vi "Shutdown.vi"(8 "Error In":errorcluster, 11 "libssh2-lv Shared Library":path=path "") -> (0 "Error Out":errorcluster)   [LabVIEW 2017, in "Toolkit.lvlib"]
uses:
  Toolkit.lvlib
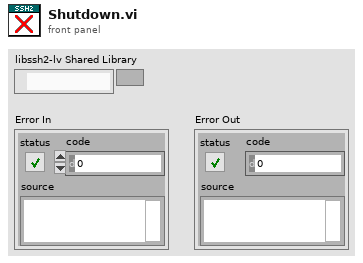
[diagram p1: front panel]
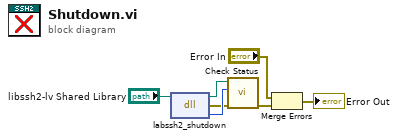
[diagram p0: block diagram]
diagram:
  n1 = dll-call lib="D:/Users/cfield/Code/Field R&D Services/SSH/LabSSH2/LabVIEW/trunk/src/Toolkit/Support/labssh2.*" fn="labssh2_shutdown"(path in="libssh2-lv Shared Library") -> (path out=w4:path, error out=w2:errorcluster, "return type"=w3:i32)  [unwired: 2 in]
  n2 = call "Check Status.vi"("Error In"=w2, "Status"=w3, "labssh2 Shared Library In"=w4) -> ("Error Out"=w1:errorcluster)  [unwired: 7 in, 1 out]
  n3 = Merge Errors("Error In", w1) -> (→"Error Out":errorcluster)
